vi "Change Active Sheet.vi"(8 "error in (no error)":errorcluster, 11 "workbook in":refnum<class "workbook.lvclass">) -> (0 "error out":errorcluster, 3 "workbook out":refnum<class "workbook.lvclass">)   [LabVIEW 2017, in "Excel_Specific.lvlib" / "workbook.lvclass"]
uses:
  workbook.lvclass
  Get Worksheet Names.vi
panel:
  in  "Sheet Name":string
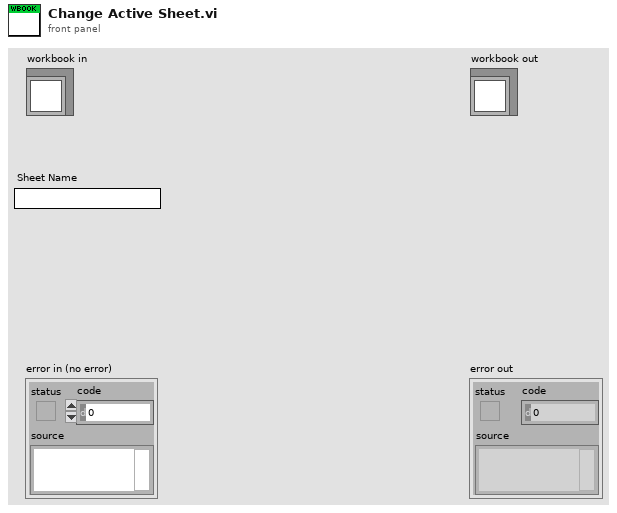
[diagram p1: front panel]
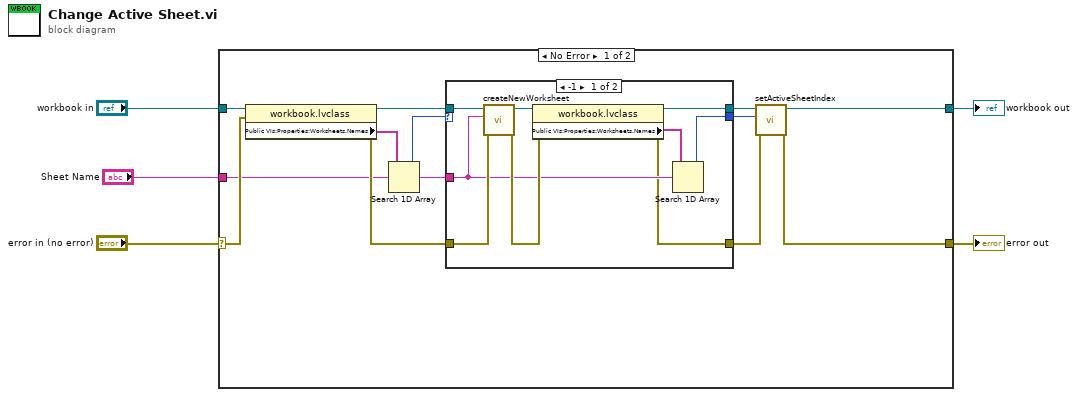
[diagram p0: block diagram]
diagram:
  n1 = case shown="No Error" "error in (no error)" {
    selector: "error in (no error)" -> [w15 w31]
    tunnel: [w6 w31] -> w4
    tunnel: [w8 w30] -> w2
    tunnel: "workbook in" -> [w16 w30]
    tunnel: "Sheet Name" -> [w11 _]
    frame No Error {
      n2 = property class="workbook.lvclass"(reference=w16, error in=w15) -> (reference out=w14:refnum<class "workbook.lvclass">, error out=w12:errorcluster, "Public VIs:Properties:Worksheets.Names"=w17:string[])
      n3 = Search 1D Array(1D array=w17, element=w11) -> (index of element=w13:i32)  [unwired: 1 in]
      n4 = case shown="-1" w13 {
        selector: w13 -> [_ w27]
        tunnel: w14 -> [w26 w29]
        tunnel: [w21 w29] -> w9
        tunnel: w12 -> [w25 w28]
        tunnel: [w18 w28] -> w7
        tunnel: w11 -> [w20 _]
        tunnel: [w19 w27] -> w10
        frame -1 {
          n5 = call "createNewWorksheet.vi"("error in (no error)"=w25, "Worksheet Name"=w20, "workbook in"=w26) -> ("error out"=w23:errorcluster, "workbook out"=w22:refnum<class "workbook.lvclass">)  [unwired: 7 in]
          n6 = property class="workbook.lvclass"(reference=w22, error in=w23) -> (reference out=w21:refnum<class "workbook.lvclass">, error out=w18:errorcluster, "Public VIs:Properties:Worksheets.Names"=w24:string[])
          n7 = Search 1D Array(1D array=w24, element=w20) -> (index of element=w19:i32)  [unwired: 1 in]
        }
        frame Default {
        }
      }
      n8 = call "setActiveSheetIndex.vi"("error in (no error)"=w7, "ActiveSheetIndex"=w10, "workbook in"=w9) -> ("error out"=w6:errorcluster, "workbook out"=w8:refnum<class "workbook.lvclass">)  [unwired: 7 in]
    }
    frame Error {
    }
  }
  "error out" <- w4
  "workbook out" <- w2
